vi "str to float.vi"(2 "String":string) -> (6 "float":sgl)   [LabVIEW 2013, in "CreateOPCUAServerAuto.lvlib"]
uses:
  CreateOPCUAServerAuto.lvlib
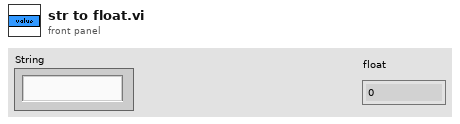
[diagram p1: front panel]
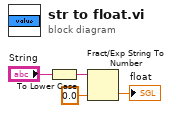
[diagram p0: block diagram]
diagram:
  n1 = To Lower Case(string="String") -> (all lower case string=w3:string)
  n2 = Fract/Exp String To Number(string=w3, default (0 dbl)=sgl 0.0 ("default (0 DBL)")) -> (number=→"float":sgl)  [unwired: 2 in, 1 out]
